vi "Import QD Shortcuts.vi"() -> ()   [LabVIEW 2012, in "NEVSTOP_QuickDrop.lvlib"]
uses:
  NEVSTOP_QuickDrop.lvlib
  user.lib/_NEVSTOP/_QuickDrop/_Support/XTwoColSelector.v1.1.llb/XTwoColumnSelector.xctl
panel:
  in  "XTwoColumnSelector":string[](xcontrol)
  in  "System OK Button":bool
  in  "System Cancel Button":bool
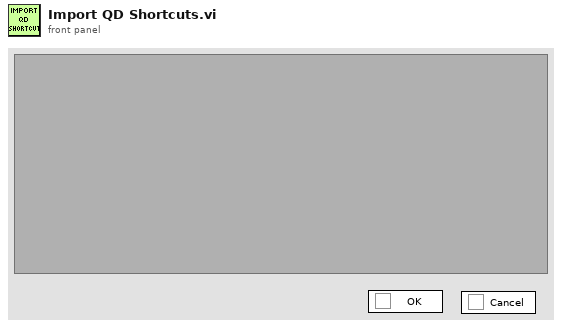
[diagram p1: front panel]
types:
  T1 = typedef "Def-IniTokenCluster.ctl" = cluster{"Session":string, "Token":string, "ListConnector":string}
  T2 = cluster{"IniTokenCluster":T1, "Items":string[]}[]
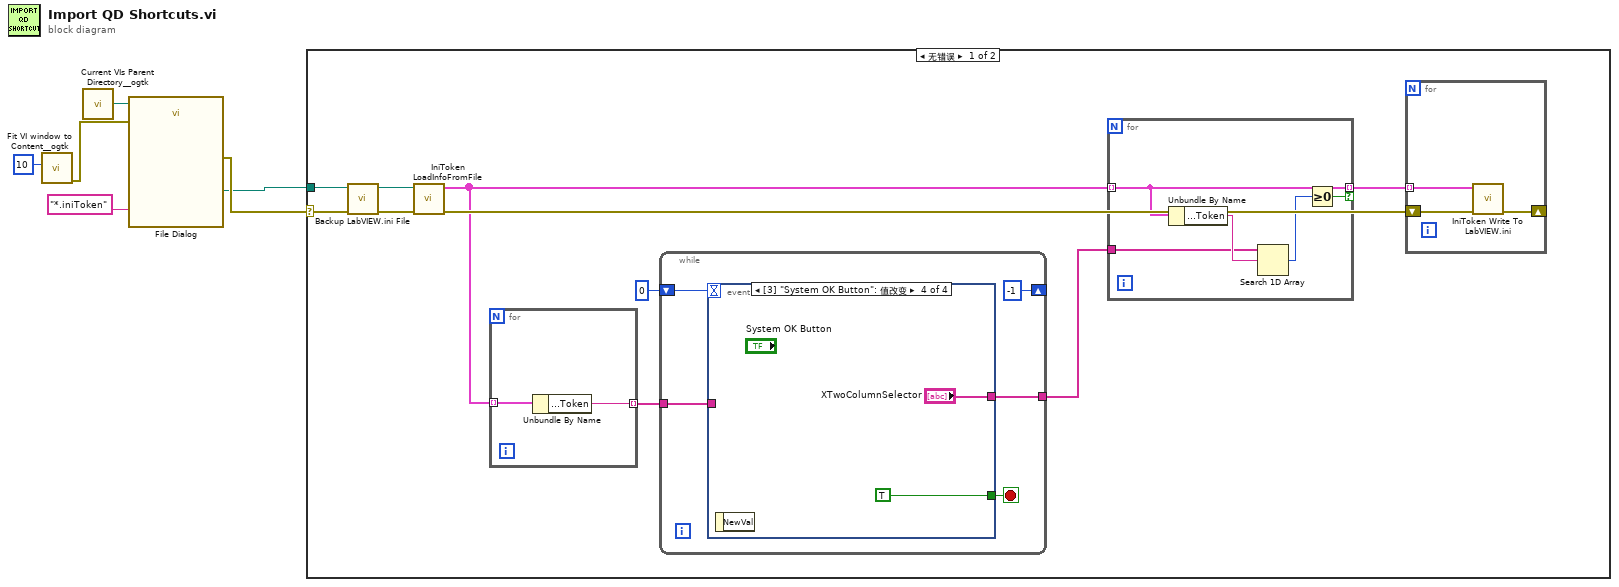
[diagram p0: block diagram]
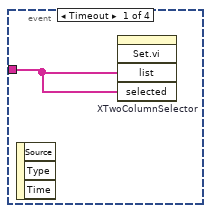
[diagram p2: hidden frame]
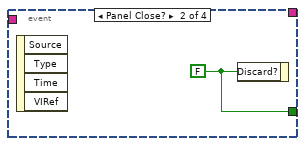
[diagram p3: hidden frame]
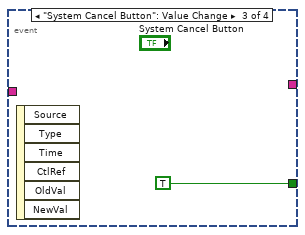
[diagram p4: hidden frame]
diagram:
  n1 = call <userlib>:"Fit VI window to Content__ogtk.vi"("border spacing (2 px)"=10) -> ("error out"=w3:errorcluster)  [unwired: 5 in, 1 out]
  n2 = call <userlib>:"Current VIs Parent Directory__ogtk.vi"() -> ("Parent Directory (+ Relative)"=w4:path)  [unwired: 5 in]
  n3 = call "File Dialog"("start path"=w4, "error in"=w3, "pattern (all files)"="*.iniToken") -> ("selected path"=w1:path, "error out"=w5:errorcluster)  [unwired: 9 in, 2 out]
  n4 = case shown="无错误" w5 {
    selector: w5 -> [w13 _]
    tunnel: w1 -> [w14 _]
    frame No Error {
      n5 = call "Backup LabVIEW.ini File.vi"("error in (no error)"=w13) -> ("error out"=w7:errorcluster)  [unwired: 9 in, 1 out]
      n6 = call "IniToken LoadInfoFromFile.vi"("error in (no error)"=w7, "Path"=w14) -> ("error out"=w12:errorcluster, "Array"=w10:T2)  [unwired: 8 in]
      n7 = for {
        tunnel: w10 -> [w22] mode=indexing
        tunnel: [w21] -> w11 mode=indexing
        n8 = Unbundle By Name(w22) -> ("IniTokenCluster.Token"=w21:string)
      }
      n9 = while {
        tunnel: [w29] -> w8
        shift-right: [-1] -> _
        shift-left: 0 -> [w28]
        tunnel: w11 -> [w26]
        stop <- w30 stop-if-true
        n10 = event shown="[3] \"System OK Button\": 值改变" {
          selector: _ -> [_ _ _ _]
          dyn-events: _ -> [_ _ _ _]
          timeout: w28 -> [_ _ _ _]
          tunnel: [_ w32 TRUE ("Discard?") TRUE ("Discard?")] -> w30
          tunnel: [_ _ _ "XTwoColumnSelector"] -> w29
          tunnel: w26 -> [w31 _ _ _]
          event Timeout {
            n11 = event-data() -> ()  [unwired: 1 in, 3 out]
            n12 = invoke on="XTwoColumnSelector" class="XTwoColumnSelector (strict)" method="Set.vi"("list"=w31, "selected"=w31) -> ()  [unwired: 3 in, 5 out]
          }
          event Panel Close? {
            w32 = FALSE ("Discard?")
            n13 = event-data() -> ()  [unwired: 1 in, 4 out]
            n14 = event-data("Discard?"=w32) -> ()  [unwired: 1 in, 1 out]
          }
          event "System Cancel Button": Value Change {
            n15 = event-data() -> ()  [unwired: 1 in, 6 out]
          }
          event "System OK Button": Value Change {
            n16 = event-data() -> ()  [unwired: 1 in, 1 out]
          }
        }
      }
      n17 = for {
        tunnel: w10 -> [w20] mode=indexing
        tunnel: [w20] -> w9 mode=indexing if=w16
        tunnel: w8 -> [w18]
        n18 = Unbundle By Name(w20) -> ("IniTokenCluster.Token"=w19:string)
        n19 = Search 1D Array(1D array=w18, element=w19) -> (index of element=w17:i32)  [unwired: 1 in]
        n20 = Greater Or Equal To 0?(x=w17) -> (x >= 0?=w16:bool)
      }
      n21 = for {
        tunnel: w9 -> [w25] mode=indexing
        shift-right: [w23] -> _
        shift-left: w12 -> [w24]
        n22 = call "IniToken Write To LabVIEW.ini.vi"("error in (no error)"=w24, "Cluster"=w25) -> ("error out"=w23:errorcluster)  [unwired: 9 in]
      }
    }
    frame Error {
    }
  }
